vi "Calculate Pixel Size.vi"(8 "error in":errorcluster, 11 "Physical Image in":T1) -> (0 "error out":errorcluster, 1 "Pixel Size y(mm)":dbl, 2 "Pixel Size x(mm)":dbl, 3 "Physical Image Out":T1)   [LabVIEW 2023]
uses:
  Type Definitions/Physical Image.ctl
  Vec3d Class/Vec3d.lvclass
  <vilib>/vision/Image Controls.llb/IMAQ Image.ctl
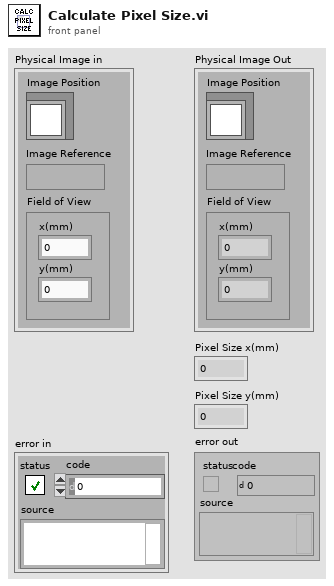
[diagram p1: front panel]
types:
  T1 = typedef "Physical Image.ctl" = cluster{"Image Position":refnum<class "Vec3d.lvclass">, "Image Reference":T2, "Field of View":cluster{"x(mm)":dbl, "y(mm)":dbl}}
  T2 = typedef "IMAQ Image.ctl" = refnum<image>
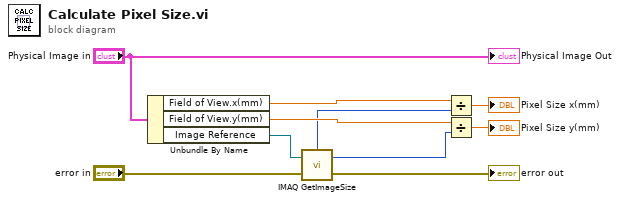
[diagram p0: block diagram]
diagram:
  n1 = Unbundle By Name("Physical Image in") -> ("Field of View.x(mm)"=w7:dbl, "Field of View.y(mm)"=w6:dbl, "Image Reference"=w9:T2)
  n2 = call "IMAQ GetImageSize"("Image"=w9, "error in (no error)"="error in") -> ("Y Resolution"=w4:i32, "X Resolution"=w5:i32, "error out"=→"error out":errorcluster)  [unwired: 2 in]
  n3 = Divide(x=w7, y=w5) -> (x/y=→"Pixel Size x(mm)":dbl)
  n4 = Divide(x=w6, y=w4) -> (x/y=→"Pixel Size y(mm)":dbl)
  "Physical Image Out" <- "Physical Image in"
